vi "cRIO_4DoF_Yaw_mouse2global_v2.vi"(10 "yawangle":dbl, 11 "Mouse forces":dbl[](array[numeric])) -> (3 "F_2":dbl[](array[numeric]))   [LabVIEW 2019]
uses:
  <vilib>/imath/engines/lvmath2/RunTimeEngine/Managers/WorkSpace/UID Generator.vi
  <vilib>/imath/engines/lvmath2/RunTimeEngine/BuiltInFunctions/size/NIMS_[I32,I32]=size(GRow).vi
  <instcachedir>/0/NIMS_[I32,I32]=size(GRow)_CFE2C4BDC5BC45CD88F2F6A295A2273D.lvgen/NIMS_[I32,I32]=size(GRow)_CFE2C4BDC5BC45CD88F2F6A295A2273D_001.vi
  <vilib>/imath/engines/lvmath2/RunTimeEngine/RunTimeType/NIMS_RunTimeType_From StrictType (excl LVString).vi
  <instcachedir>/0/NIMS_RunTimeType_From StrictType (excl LVString)_D8AFBA86A94845AAA577C895450664BD.lvgen/NIMS_RunTimeType_From StrictType (excl LVString)_D8AFBA86A94845AAA577C895450664BD_000.vi
  <vilib>/imath/engines/lvmath2/RunTimeEngine/LocalVariableDefStatement/MC_LocalVariableDefStatement_Display.vi
  <vilib>/imath/engines/lvmath2/RunTimeEngine/IndexRead/NIMS M(R2,S).vi
  <instcachedir>/0/NIMS M(R2,S)_56813DCFDD5A484292D2195AF15D2BF5.lvgen/NIMS M(R2,S)_56813DCFDD5A484292D2195AF15D2BF5_000.vi
  <vilib>/imathl/engines/lvmath/Functions/Error Handling/Create Error.vi
  <vilib>/imath/engines/lvmath2/RunTimeEngine/ArithmeticOperatorToken/NIMS_ArithmeticOperator_multmx(M,CV)-internal.vi
  <instcachedir>/0/NIMS_ArithmeticOperator_multmx(M,CV)-internal_2C55777844884EEDB828A940D397C7D0.lvgen/NIMS_ArithmeticOperator_multmx(M,CV)-internal_2C55777844884EEDB828A940D397C7D0_001.vi
  <vilib>/imath/engines/lvmath2/RunTimeEngine/IndexRead/NIMS M(S,S).vi
  <instcachedir>/0/NIMS M(S,S)_AC51E74150A542F7991B9634C66F3096.lvgen/NIMS M(S,S)_AC51E74150A542F7991B9634C66F3096_000.vi
  <vilib>/imath/engines/lvmath2/RunTimeEngine/Managers/SymbolTable/Clear UID.vi
  <vilib>/imath/engines/lvmath2/RunTimeEngine/NodeEndStatement/NIMS_NodeEndStatement_Output.vi
  <instcachedir>/0/NIMS_NodeEndStatement_Output_53EC0D466D134D7ABD903AC30B43404B.lvgen/NIMS_NodeEndStatement_Output_53EC0D466D134D7ABD903AC30B43404B_005.vi
  <vilib>/imath/engines/lvmath2/RunTimeEngine/ErrorHandling/NIMS_Finalize Error.vi
  <vilib>/imath/engines/lvmath2/RunTimeEngine/Managers/SymbolTable/NIMS_WorkSpace.lvlib
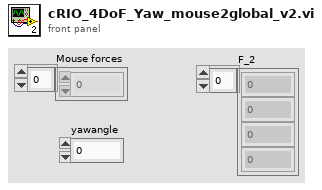
[diagram p1: front panel]
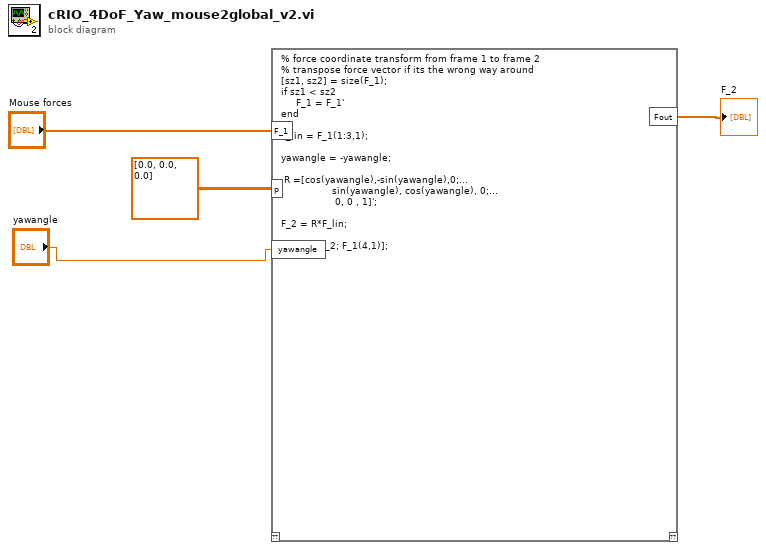
[diagram p0: block diagram]
diagram:
  n1 = mathscript code="% force coordinate transform from frame 1 to frame 2 \n% transpose force vector if its the wrong way around\n[sz1, sz2] = size(F_1);\nif sz1 < sz2\n     F_1 = F_1'\nend\n\nF_lin = F_1(1:3,1);\n\nyawangle = -yawangle; \n\n R =[cos(yawangle),-sin(yawangle),0;...\n                 sin(yawangle), cos(yawangle), 0;...\n                  0, 0 , 1]';\n\nF_2 = R*F_lin;\n\nFout = [F_2; F_1(4,1)];"("F_1"="Mouse forces", "p"=dbl[][] [[0.0], [0.0], [0.0]], "yawangle"="yawangle") -> ("Fout"=→"F_2":dbl[])  [unwired: 1 in, 1 out]
